vi "compress_tiff_example.vi"() -> ()   [LabVIEW 2020]
panel:
  out "dp_status_init":i32
  in  "path to TIFF file":path
  out "dp_status_prepare":i32
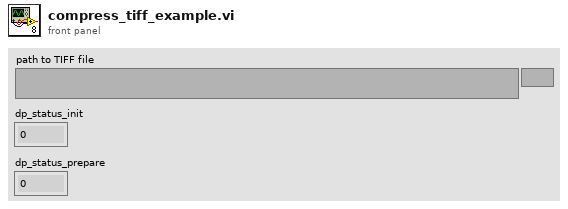
[diagram p1: front panel]
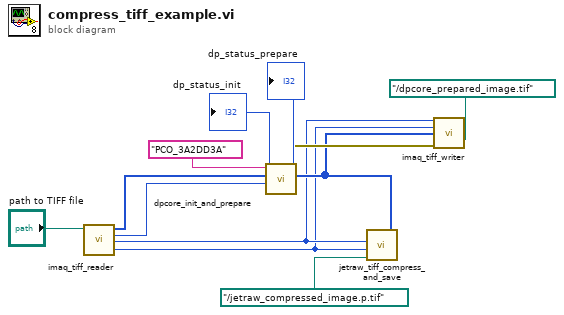
[diagram p0: block diagram]
diagram:
  n1 = call "imaq_tiff_reader.vi"("path to TIFF file"="path to TIFF file") -> ("image_height"=w2:i32, "image_width"=w3:i32, "image_buffer (U16)"=w11:u16[], "image_length"=w7:i32)  [unwired: 7 in]
  n2 = call "dpcore_init_and_prepare.vi"("image_length"=w7, "Image Pixels (U16)"=w11, "identifier"="PCO_3A2DD3A" ("file_path")) -> ("error out"=w6:errorcluster, "dp_status_prepare"=→"dp_status_prepare":i32, "prepared_image_buffer"=w4:u16[], "dp_status_init"=→"dp_status_init":i32)  [unwired: 5 in]
  n3 = call "jetraw_tiff_compress_and_save.vi"("compressed output filename"=path "../jetraw_compressed_image.p.tif" ("name or relative path"), "height"=w2, "width"=w3, "image_buffer"=w4) -> ()  [unwired: 8 in]
  n4 = call "imaq_tiff_writer.vi"("image_width"=w3, "image_height"=w2, "output_buffer in"=w4, "name or relative path"=path "../dpcore_prepared_image.tif", "error in (no error)"=w6) -> ()  [unwired: 11 in]
